vi "Pre Launch Init.vi"(11 "Publisher Actor in":refnum<class "Publisher Actor.lvclass">) -> (0 "error out":errorcluster, 3 "Publisher Actor out":refnum<class "Publisher Actor.lvclass">)   [LabVIEW 2021, in "Publisher Actor.lvclass"]
doc: "(<B>Filename</B>: Actor Framework.lvlib:Actor.lvclass:Pre Launch Init.vi)\n\nDefines behavior that occurs after the Launch Nested Actor method is invoked but before the actor's Actor Core method begins running.\n\nBy default, this method does nothing. A descendant class may override it to define behavior."
uses:
  Publisher Actor.lvclass
  Context.ctl
  <vilib>/ActorFramework/Message Enqueuer/Message Enqueuer.lvclass
  Publisher Actor.lvclass/Publisher Actor.ctl
  <vilib>/ActorFramework/Actor/Actor.lvclass
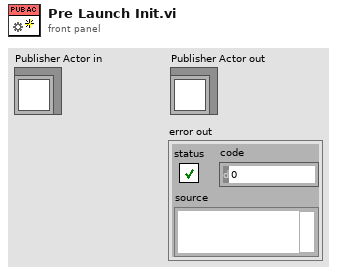
[diagram p1: front panel]
types:
  T1 = typedef "Context.ctl" = cluster{"Topic":string, "Source":string}
  T2 = map{T1, set{refnum<class "Message Enqueuer.lvclass">}}
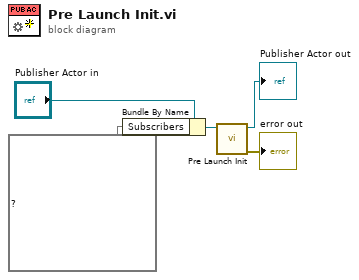
[diagram p0: block diagram]
diagram:
  n1 = Bundle By Name(cluster="Publisher Actor in", "Subscribers"=T2 {}) -> (w2:refnum<class "Publisher Actor.lvclass">)
  n2 = call-parent "Pre Launch Init.vi"("Actor in"=w2) -> ("error out"=→"error out":errorcluster, "Actor out"=→"Publisher Actor out":refnum<class "Publisher Actor.lvclass">)  [unwired: 9 in]
